vi "write_to_logfile.vi"(7 "Test vector":T1, 8 "error in (no error)":errorcluster, 9 "Array":T9[](array[typedef]), 10 "Test sequence results":T6 {"Time Stamp" format="%<%.3X>T"}, 11 "Log file":path) -> (0 "error out":errorcluster)   [LabVIEW 2024]
doc: "Writes Test vector, Test sequence results and Output Array types into a text formatted log file defined by its path."
uses:
  ctl_test_outputs_cluster.ctl
  ctl_results_array.ctl
  ctl_results_cluster.ctl
  ctl_pass_fail_led.ctl
  ctl_test_vector_array.ctl
  ctl_test_item_cluster.ctl
  ctl_stimuli_cluster.ctl
  ctl_loads_enum.ctl
  ctl_pass_limits_cluster.ctl
  <vilib>/Utility/file.llb/Write Delimited Spreadsheet (DBL).vi
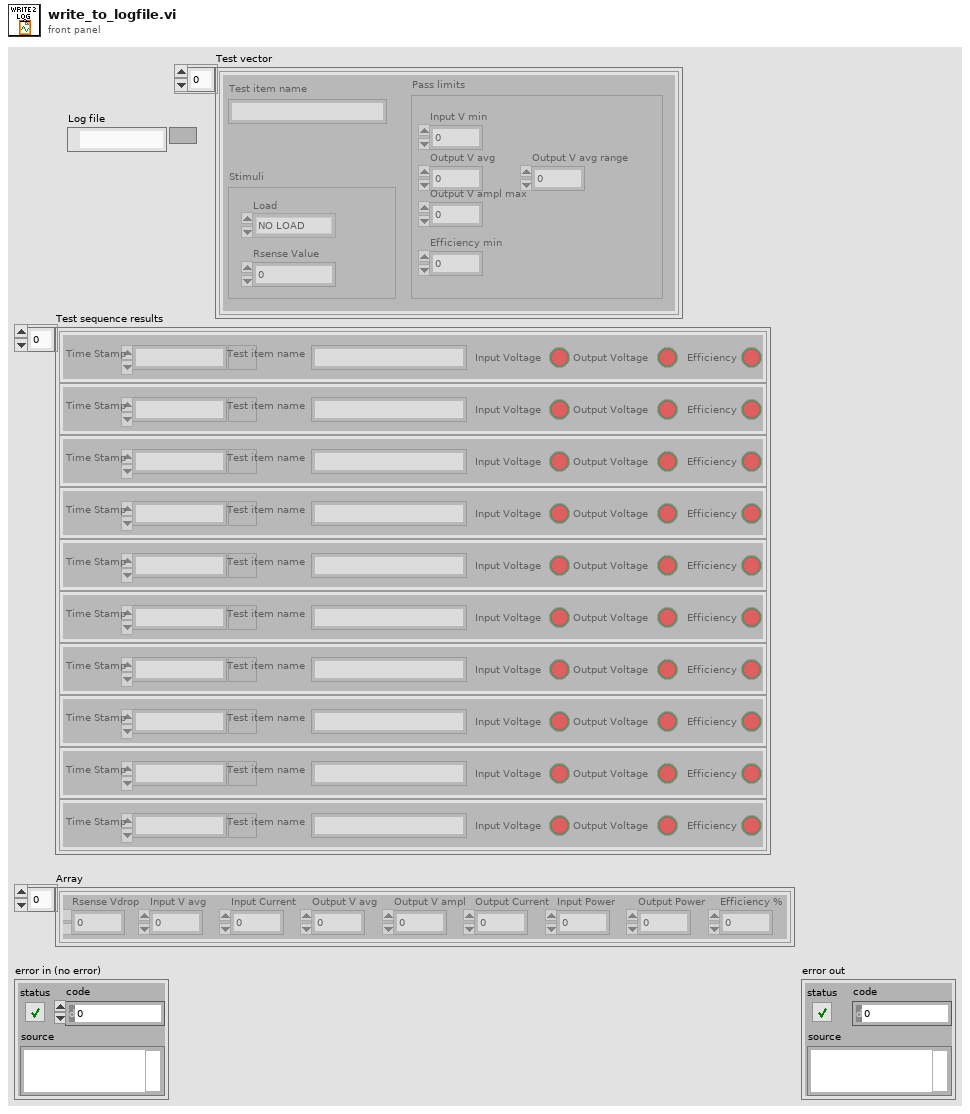
[diagram p1: front panel]
types:
  T1 = typedef "ctl_test_vector_array.ctl" = T2[]
  T2 = typedef "ctl_test_item_cluster.ctl" = cluster{"Stimuli":T3, "Pass limits":T5, "Test item name":string}
  T3 = typedef "ctl_stimuli_cluster.ctl" = cluster{"Load":T4, "Rsense Value":dbl}
  T4 = typedef "ctl_loads_enum.ctl" = enum16{"NO LOAD", "10Ohm", "6.8Ohm", "4.7Ohm", "3.3Ohm", "2.4Ohm", "1.6Ohm", "1.3Ohm"}
  T5 = typedef "ctl_pass_limits_cluster.ctl" = cluster{"Output V avg":dbl, "Output V ampl max":dbl, "Efficiency min":dbl, "Input V min":dbl, "Output V avg range":dbl}
  T6 = typedef "ctl_results_array.ctl" = T7[]
  T7 = typedef "ctl_results_cluster.ctl" = cluster{"Time Stamp":timestamp, "Test item name":string, "Input Voltage":T8, "Output Voltage":T8, "Efficiency":T8}
  T8 = typedef "ctl_pass_fail_led.ctl" = bool
  T9 = typedef "ctl_test_outputs_cluster.ctl" = cluster{"Output V avg":dbl, "Output V ampl":dbl, "Input Current":dbl, "Output Current":dbl, "Efficiency %":dbl, "Input V avg":dbl, "Input Power":dbl, "Output Power":dbl, "Rsense Vdrop":dbl}
  T10 = enum16{"open", "replace", "create", "open or create", "replace or create", "replace or create with confirmation"}
  T11 = typedef "ctl_meas_env_cluster.ctl" = cluster{"Rsense_value Ohm":dbl, "Rload_value Ohm":dbl}
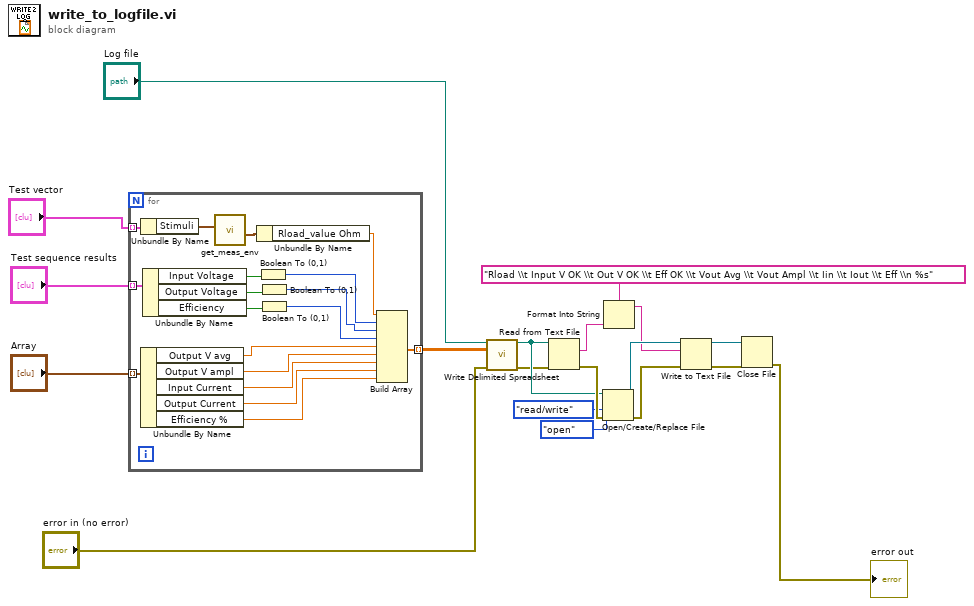
[diagram p0: block diagram]
diagram:
  n1 = for {
    tunnel: "Test sequence results" -> [w37] mode=indexing
    tunnel: "Array" -> [w36] mode=indexing
    tunnel: [w24] -> w4 mode=indexing
    tunnel: "Test vector" -> [w23] mode=indexing
    n2 = Unbundle By Name(w23) -> ("Stimuli"=w22:T3)
    n3 = Unbundle By Name(w36) -> ("Output V avg"=w29:dbl, "Output V ampl"=w28:dbl, "Input Current"=w27:dbl, "Output Current"=w26:dbl, "Efficiency %"=w25:dbl)
    n4 = Unbundle By Name(w37) -> ("Input Voltage"=w35:T8, "Output Voltage"=w34:T8, "Efficiency"=w33:T8)
    n5 = call "get_meas_env.vi"("Stimuli"=w22) -> ("Meas environment"=w21:T11)  [unwired: 9 in, 1 out]
    n6 = Unbundle By Name(w21) -> ("Rload_value Ohm"=w20:dbl)
    n7 = Boolean To (0,1)(Boolean=w35) -> (0, 1=w32:i16)
    n8 = Boolean To (0,1)(Boolean=w34) -> (0, 1=w31:i16)
    n9 = Boolean To (0,1)(Boolean=w33) -> (0, 1=w30:i16)
    n10 = Build Array(w20, w32, w31, w30, w29, w28, w27, w26, w25) -> (w24:dbl[])
  }
  n11 = call-poly <vilib>:"Write Delimited Spreadsheet.vi"("file path (dialog if empty)"="Log file", "2D data"=w4, "error in (no error)"="error in (no error)") -> ("new file path (Not A Path if cancelled)"=w10:path, "error out"=w7:errorcluster)  [unwired: 11 in]
  n12 = Read from Text File(file (use dialog)=w10, error in=w7) -> (text=w8:string, error out=w13:errorcluster)  [unwired: 2 in, 2 out]
  n13 = Open/Create/Replace File(file path (use dialog)=w10, error in=w13, operation (0:open)=T10."open", access (0:read/write)=enum16{"read/write", "read-only", "write-only"}."read/write") -> (refnum out=w15:refnum<file>, error out=w14:errorcluster)  [unwired: 2 in, 1 out]
  n14 = Format Into String(format string="Rload \\t Input V OK \\t Out V OK \\t Eff OK \\t Vout Avg \\t Vout Ampl \\t Iin \\t Iout \\t Eff \\n %s", w8) -> (resulting string=w9:string)  [unwired: 2 in, 1 out]
  n15 = Write to Text File(file (use dialog)=w15, text=w9, error in=w14) -> (refnum out=w17:refnum<file>, error out=w16:errorcluster)  [unwired: 1 in, 1 out]
  n16 = Close File(refnum=w17, error in=w16) -> (error out=→"error out":errorcluster)  [unwired: 1 out]
